vi "BuildTree.vi"(10 "appended path":path, 11 "TreeControl in":refnum<vi>) -> ()   [LabVIEW 2016]
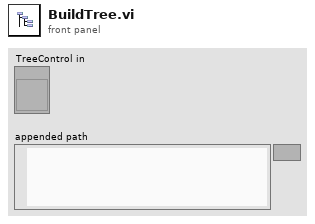
[diagram p1: front panel]
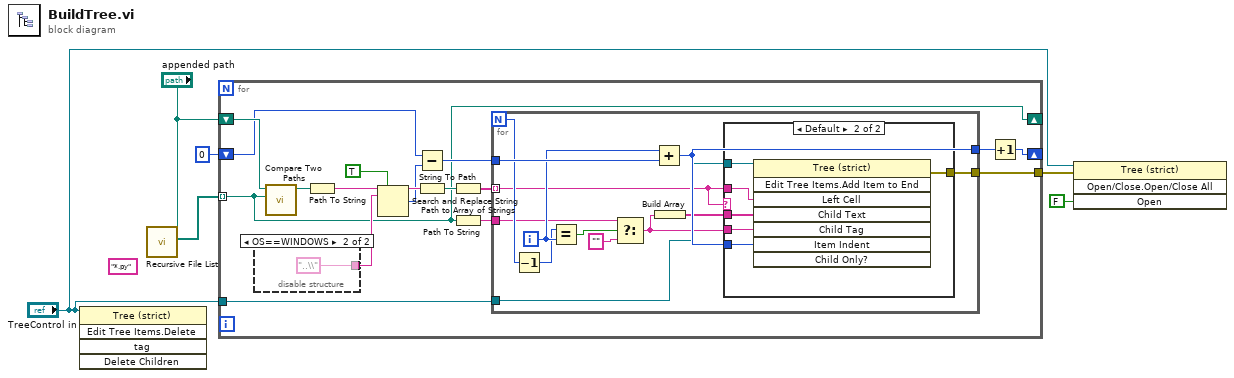
[diagram p0: block diagram]
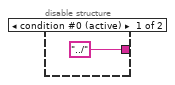
[diagram p2: hidden frame]
diagram:
  (unwired) "*.py" ("pattern")
  n1 = invoke on="Invoke Node" class="Tree (strict)" method="Edit Tree Items.Delete"(reference="TreeControl in") -> ()  [unwired: 4 in, 5 out]
  n2 = call <vilib>:"Recursive File List.vi"("Folder Path"="appended path") -> ("All Files in Dir"=w4:path[])  [unwired: 6 in, 4 out]
  n3 = for {
    tunnel: w4 -> [w10] mode=indexing
    shift-right: [w10] -> _
    shift-left: "appended path" -> [w23]
    shift-right: [w11] -> _
    shift-left: 0 -> [w13]
    tunnel: [w8] -> w2
    tunnel: "TreeControl in" -> [w7]
    n4 = disable-structure shown="OS==WINDOWS" {
      disable-tunnel: ["../" ("search string") "..\\" ("search string")] -> w21
      frame condition #0 (active) {
      }
      frame condition #1 {
      }
    }
    n5 = call <vilib>:"Compare Two Paths.vi"("Path 2"=w10, "Path 1"=w23) -> ("Relative Path from 1 to 2"=w15:path)  [unwired: 6 in, 3 out]
    n6 = Path To String(path=w15) -> (string=w22:string)
    n7 = Search and Replace String(replace all?=TRUE ("replace all? (F)"), input string=w22, search string=w21) -> (result string=w19:string, number of replacements=w16:i32)  [unwired: 5 in, 2 out]
    n8 = Subtract(x=w13, y=w16) -> (x-y=w14:i32)
    n9 = String To Path(string=w19) -> (path=w18:path)
    n10 = Path to Array of Strings(0:w18) -> (2:w17:string[])  [unwired: 1 out]
    n11 = Path To String(path=w10) -> (string=w9:string)
    n12 = for {
      N -> [w35]
      tunnel: w17 -> [w26] mode=indexing
      tunnel: w14 -> [w38]
      tunnel: [w37] -> w12
      tunnel: w9 -> [w29]
      tunnel: [w28] -> w8
      tunnel: w7 -> [w27]
      i -> [w36]
      n13 = Decrement(x=w35) -> (x-1=w34:i32)
      n14 = Equal?(x=w34, y=w36) -> (x = y?=w33:bool)
      n15 = Select(t=w29, s=w33, f="") -> (s? t:f=w31:string)
      n16 = Add(x=w36, y=w38) -> (x+y=w37:i32)
      n17 = Build Array(w31) -> (w30:string[])
      n18 = case shown="Default" w26 {
        tunnel: w26 -> [_ w44]
        tunnel: w37 -> [_ w43]
        tunnel: w31 -> [_ w42]
        tunnel: w30 -> [_ w41]
        tunnel: [_ w40] -> w28
        tunnel: w27 -> [_ w39]
        frame ".DS_Store" {
        }
        frame Default {
          n19 = invoke on="Invoke Node" class="Tree (strict)" method="Edit Tree Items.Add Item to End"(reference=w39, "Left Cell"=w44, "Child Text"=w41, "Child Tag"=w42, "Item Indent"=w43) -> (error out=w40:errorcluster)  [unwired: 3 in, 7 out]
        }
      }
    }
    n20 = Increment(x=w12) -> (x+1=w11:i32)
  }
  n21 = invoke on="Invoke Node" class="Tree (strict)" method="Open/Close.Open/Close All"(reference="TreeControl in", error in=w2, "Open"=FALSE ("Open?")) -> ()  [unwired: 1 in, 4 out]
